vi "FIR_stage_1.vi"(8 "data valid in":bool, 9 "Q in":fxp<+/-,16,14>[](array[numeric])=[0.0, 0.0, 0.0, 0.0], 10 "I in":fxp<+/-,16,14>[](array[numeric])=[0.0, 0.0, 0.0, 0.0]) -> (0 "data valid out":bool, 1 "Q out":fxp<+/-,16,14>, 2 "I out":fxp<+/-,16,14>)   [LabVIEW 2013]
uses:
  <vilib>/rvi/FXPMathLib/FxpConvert/subVIs/nifxpmath_Convert_SimConfig.ctl
  <vilib>/fxp/LVFixedPointQuantizationPolicyTypeDef.ctl
  <vilib>/fxp/LVFixedPointOverflowPolicyTypeDef.ctl
  <vilib>/rvi/FXPMathLib/FxpConvert/simVIs/DllFxpConvertTemp_sub.vi
  <vilib>/rvi/IPIntegrationNode/IPINode_Utilities/niFpgaIPINodeSimCore.vi
  <vilib>/rvi/FXPMathLib/FxpInterpret/XNode/nifxpmath_Interpret.xnode
  <vilib>/rvi/FXPMathLib/FxpConvert/XNode/nifxpmath_Convert.xnode
  <vilib>/rvi/FXPMathLib/FxpAdd/XNode/nifxpmath_Add.xnode
  <vilib>/rvi/XilinxIP/XIPIN_XNode/niFpgaXIPIN.xnode
  Filters/Polyphase filterbank/Filter1/Polyphase_filterbank_Filter1_C3D6D94C538F4B69A671231CBB16BC71.dll
  <vilib>/rvi/IPIntegrationNode/IPINode_Xnode/niFpgaIPINode.xnode
  Filters/Polyphase filterbank/Filter2/Polyphase_filterbank_Filter2_600B6E97182E42B4ACFE8408F669A62F.dll
  Filters/Polyphase filterbank/Filter3/Polyphase_filterbank_Filter3_90A56C0CA55345308F9FA6BEDF7A9824.dll
  Filters/Polyphase filterbank/Filter0/Polyphase_filterbank_Filter0_75806FB194E14CD7BE90987543D5A2F6.dll
  <vilib>/rvi/FXPMathLib/sim/FxpSim.dll
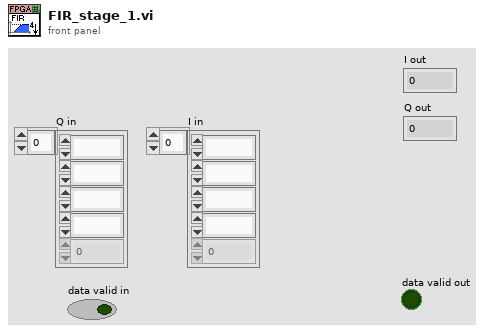
[diagram p1: front panel]
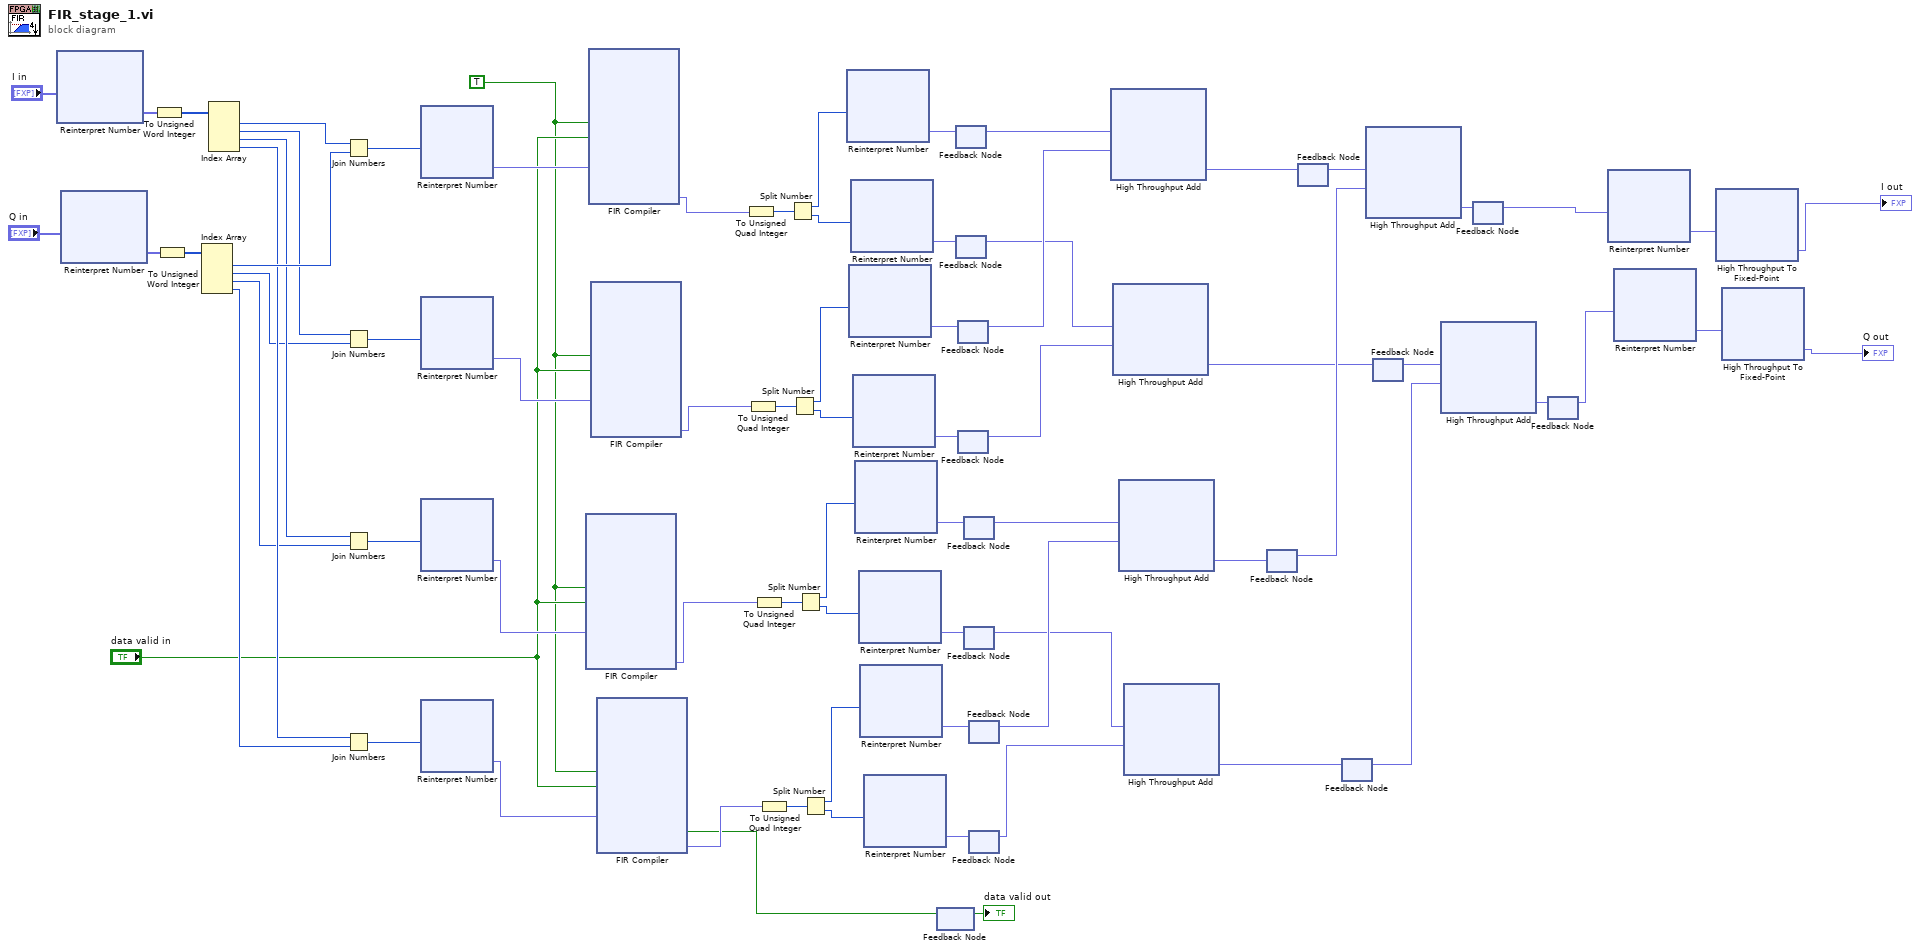
[diagram p0: block diagram]
diagram:
  w5 = TRUE ("aresetn")
  n1 = xnode "Reinterpret Number"("x"="I in") -> ("y"=w21:fxp<+,16,16>[])
  n2 = xnode "Reinterpret Number"("x"="Q in") -> ("y"=w23:fxp<+,16,16>[])
  n3 = To Unsigned Word Integer(number=w21) -> (unsigned 16bit integer=w74:u16[])
  n4 = To Unsigned Word Integer(number=w23) -> (unsigned 16bit integer=w20:u16[])
  n5 = Index Array(array=w20) -> (element #1=w72:u16, element #2=w44:u16, element #3=w43:u16, element #4=w42:u16)  [unwired: 4 in]
  n6 = Index Array(array=w74) -> (element #1=w73:u16, element #2=w47:u16, element #3=w46:u16, element #4=w45:u16)  [unwired: 4 in]
  n7 = Join Numbers(hi=w73, lo=w72) -> ((hi.lo)=w71:u32)
  n8 = Join Numbers(hi=w47, lo=w44) -> ((hi.lo)=w50:u32)
  n9 = Join Numbers(hi=w46, lo=w43) -> ((hi.lo)=w49:u32)
  n10 = Join Numbers(hi=w45, lo=w42) -> ((hi.lo)=w48:u32)
  n11 = xnode "Reinterpret Number"("x"=w71) -> ("y"=w11:fxp<+,32,32>)
  n12 = xnode "Reinterpret Number"("x"=w50) -> ("y"=w9:fxp<+,32,32>)
  n13 = xnode "Reinterpret Number"("x"=w49) -> ("y"=w8:fxp<+,32,32>)
  n14 = xnode "Reinterpret Number"("x"=w48) -> ("y"=w7:fxp<+,32,32>)
  n15 = xnode ("FIR Compiler")("aresetn"=w5, "s_axis_data_tvalid"="data valid in", "s_axis_data_tdata"=w8) -> ("m_axis_data_tdata"=w2:fxp<+,64,64>)  [unwired: 1 in, 2 out]
  n16 = xnode ("FIR Compiler")("aresetn"=w5, "s_axis_data_tvalid"="data valid in", "s_axis_data_tdata"=w11) -> ("m_axis_data_tdata"=w10:fxp<+,64,64>)  [unwired: 1 in, 2 out]
  n17 = xnode ("FIR Compiler")("aresetn"=w5, "s_axis_data_tvalid"="data valid in", "s_axis_data_tdata"=w9) -> ("m_axis_data_tdata"=w1:fxp<+,64,64>)  [unwired: 1 in, 2 out]
  n18 = xnode ("FIR Compiler")("aresetn"=w5, "s_axis_data_tvalid"="data valid in", "s_axis_data_tdata"=w7) -> ("m_axis_data_tvalid"=w3:bool, "m_axis_data_tdata"=w4:fxp<+,64,64>)  [unwired: 1 in, 1 out]
  n19 = To Unsigned Quad Integer(1:w10) -> (0:w70:u64)
  n20 = To Unsigned Quad Integer(1:w1) -> (0:w60:u64)
  n21 = To Unsigned Quad Integer(1:w2) -> (0:w59:u64)
  n22 = To Unsigned Quad Integer(1:w4) -> (0:w18:u64)
  n23 = Split Number(x=w70) -> (hi(x)=w68:u32, lo(x)=w66:u32)
  n24 = Split Number(x=w60) -> (hi(x)=w61:u32, lo(x)=w63:u32)
  n25 = Split Number(x=w59) -> (hi(x)=w58:u32, lo(x)=w56:u32)
  n26 = Split Number(x=w18) -> (hi(x)=w51:u32, lo(x)=w53:u32)
  n27 = xnode "Reinterpret Number"("x"=w68) -> ("y"=w67:fxp<+/-,32,14>)
  n28 = xnode "Reinterpret Number"("x"=w61) -> ("y"=w62:fxp<+/-,32,14>)
  n29 = xnode "Reinterpret Number"("x"=w66) -> ("y"=w65:fxp<+/-,32,14>)
  n30 = xnode "Reinterpret Number"("x"=w63) -> ("y"=w64:fxp<+/-,32,14>)
  n31 = xnode "Reinterpret Number"("x"=w58) -> ("y"=w57:fxp<+/-,32,14>)
  n32 = xnode "Reinterpret Number"("x"=w56) -> ("y"=w55:fxp<+/-,32,14>)
  n33 = xnode "Reinterpret Number"("x"=w51) -> ("y"=w52:fxp<+/-,32,14>)
  n34 = xnode "Reinterpret Number"("x"=w53) -> ("y"=w54:fxp<+/-,32,14>)
  n35 = feedback #1() -> (→"data valid out":bool)  [unwired: 1 in]
  n36 = feedback-in #1(w3) -> ()
  n37 = feedback #2() -> (w69:fxp<+/-,32,14>)  [unwired: 1 in]
  n38 = feedback-in #2(w67) -> ()
  n39 = feedback #3() -> (w36:fxp<+/-,32,14>)  [unwired: 1 in]
  n40 = feedback-in #3(w65) -> ()
  n41 = feedback #4() -> (w41:fxp<+/-,32,14>)  [unwired: 1 in]
  n42 = feedback-in #4(w62) -> ()
  n43 = feedback #5() -> (w35:fxp<+/-,32,14>)  [unwired: 1 in]
  n44 = feedback-in #5(w64) -> ()
  n45 = feedback #6() -> (w40:fxp<+/-,32,14>)  [unwired: 1 in]
  n46 = feedback-in #6(w57) -> ()
  n47 = feedback #7() -> (w37:fxp<+/-,32,14>)  [unwired: 1 in]
  n48 = feedback-in #7(w55) -> ()
  n49 = feedback #8() -> (w39:fxp<+/-,32,14>)  [unwired: 1 in]
  n50 = feedback-in #8(w52) -> ()
  n51 = feedback #9() -> (w38:fxp<+/-,32,14>)  [unwired: 1 in]
  n52 = feedback-in #9(w54) -> ()
  n53 = xnode "High Throughput Add"("x"=w69, "y"=w41) -> ("x+y"=w31:fxp<+/-,19,15>)
  n54 = xnode "High Throughput Add"("x"=w36, "y"=w35) -> ("x+y"=w26:fxp<+/-,19,15>)
  n55 = xnode "High Throughput Add"("x"=w40, "y"=w39) -> ("x+y"=w30:fxp<+/-,19,15>)
  n56 = xnode "High Throughput Add"("x"=w37, "y"=w38) -> ("x+y"=w25:fxp<+/-,19,15>)
  n57 = feedback #10() -> (w34:fxp<+/-,19,15>)  [unwired: 1 in]
  n58 = feedback-in #10(w30) -> ()
  n59 = feedback #11() -> (w33:fxp<+/-,19,15>)  [unwired: 1 in]
  n60 = feedback-in #11(w31) -> ()
  n61 = feedback #12() -> (w27:fxp<+/-,19,15>)  [unwired: 1 in]
  n62 = feedback-in #12(w25) -> ()
  n63 = xnode "High Throughput Add"("x"=w33, "y"=w34) -> ("x+y"=w32:fxp<+/-,20,16>)
  n64 = feedback #13() -> (w28:fxp<+/-,19,15>)  [unwired: 1 in]
  n65 = feedback-in #13(w26) -> ()
  n66 = xnode "High Throughput Add"("x"=w28, "y"=w27) -> ("x+y"=w29:fxp<+/-,20,16>)
  n67 = feedback #14() -> (w15:fxp<+/-,20,16>)  [unwired: 1 in]
  n68 = feedback-in #14(w32) -> ()
  n69 = feedback #15() -> (w14:fxp<+/-,20,16>)  [unwired: 1 in]
  n70 = feedback-in #15(w29) -> ()
  n71 = xnode "Reinterpret Number"("x"=w15) -> ("y"=w17:fxp<+/-,20,14>)
  n72 = xnode "Reinterpret Number"("x"=w14) -> ("y"=w16:fxp<+/-,20,14>)
  n73 = xnode ("High Throughput To Fixed-Point")("x"=w17) -> ("y"=→"I out":fxp<+/-,16,14>)
  n74 = xnode ("High Throughput To Fixed-Point")("x"=w16) -> ("y"=→"Q out":fxp<+/-,16,14>)
